vi "MainControl, FSM proto.vi"() -> ()   [LabVIEW 2020]
uses:
  State.ctl
panel:
  in  "Poll temps.":bool
  out "Repoll?":bool
  out "Current time":timestamp format="%<%X>T"
  out "Loop iteration":i32
  in  "Halt all":bool
  in  "Move dist.":dbl
  in  "Move up":bool
  in  "Move right":bool
  in  "Move left":bool
  in  "Move Down":bool
  in  "Home printer":bool
  in  "Stop print":bool
  out "STATE":T1
  in  "Start print":bool
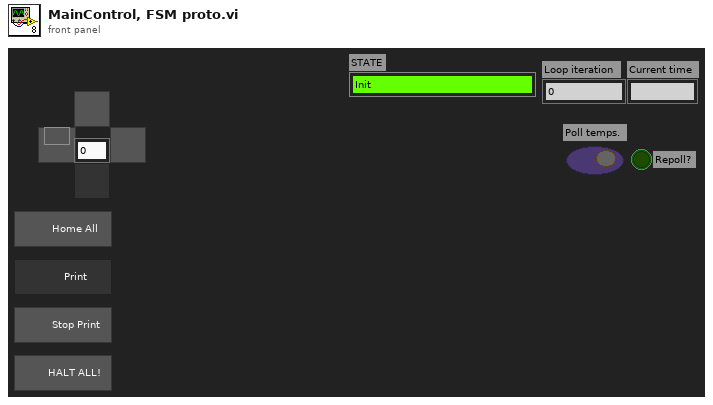
[diagram p1: front panel]
types:
  T1 = typedef "State.ctl" = enum16{"Init", "Idle", "Moving", "Printing - Container", "Printing - Curing", "Printing - Support Bath", "Printing - Biomaterial", "Stop print", "Halt all"}
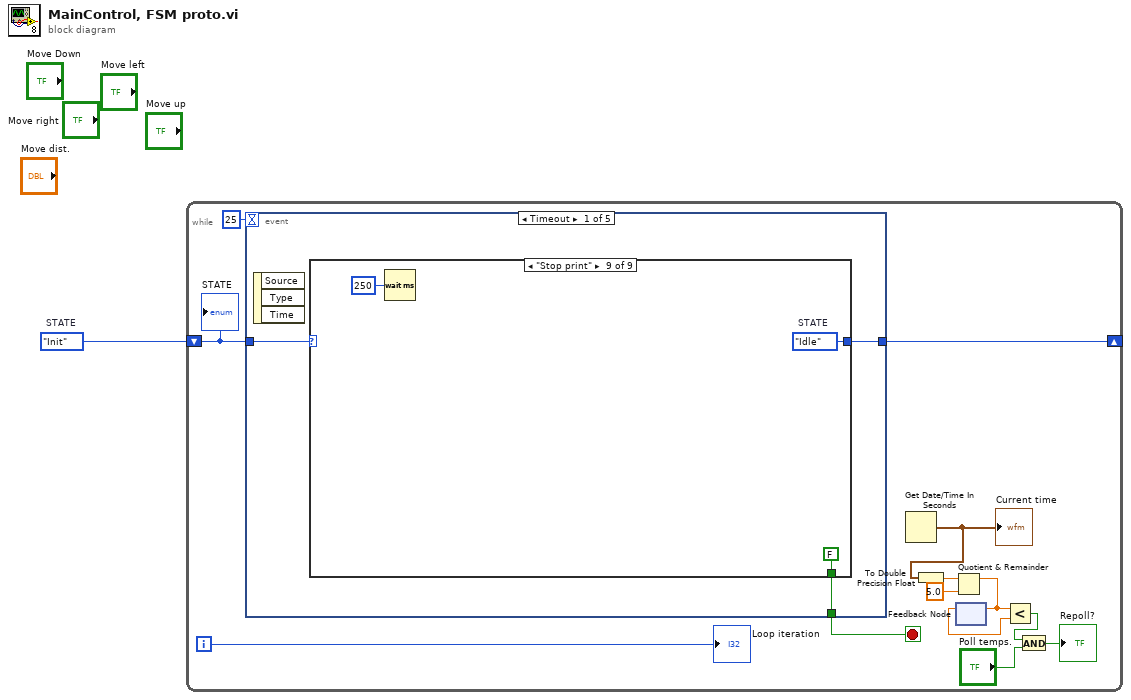
[diagram p0: block diagram]
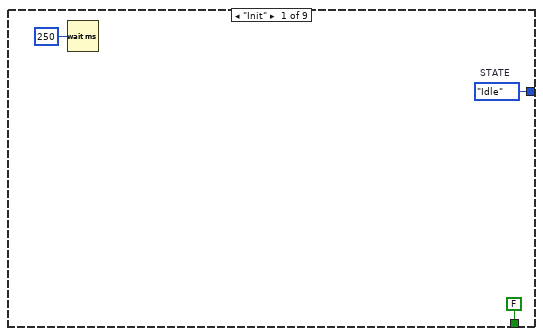
[diagram p2: hidden frame]
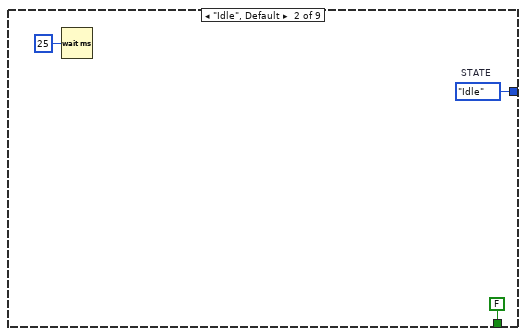
[diagram p3: hidden frame]
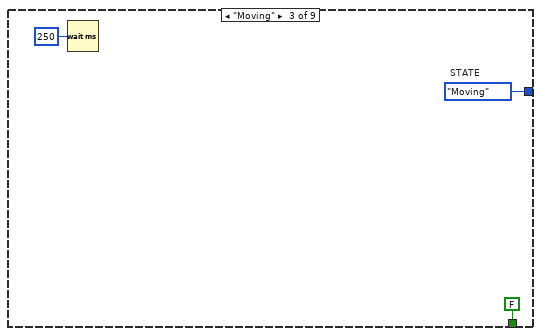
[diagram p4: hidden frame]
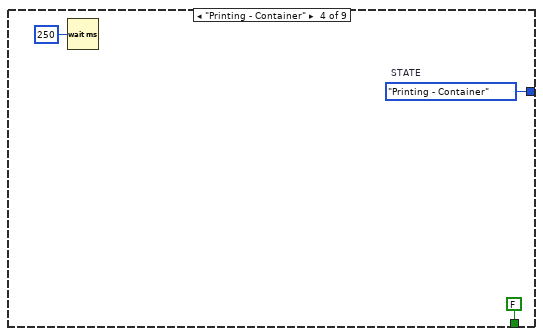
[diagram p5: hidden frame]
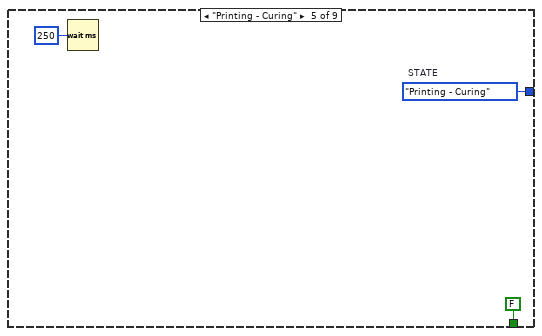
[diagram p6: hidden frame]
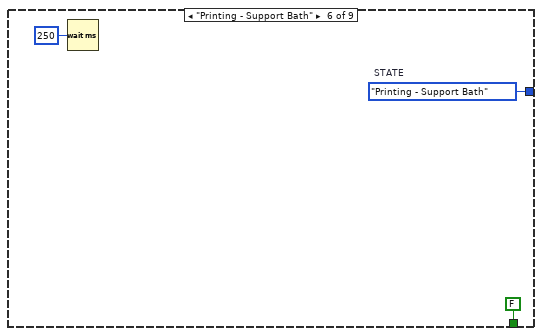
[diagram p7: hidden frame]
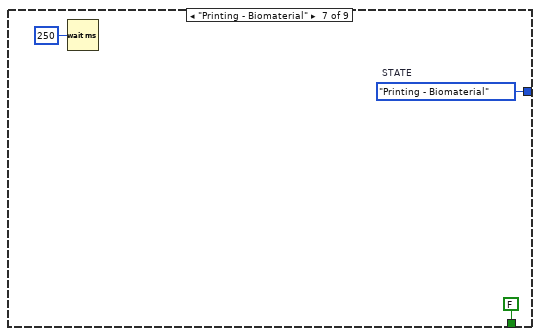
[diagram p8: hidden frame]
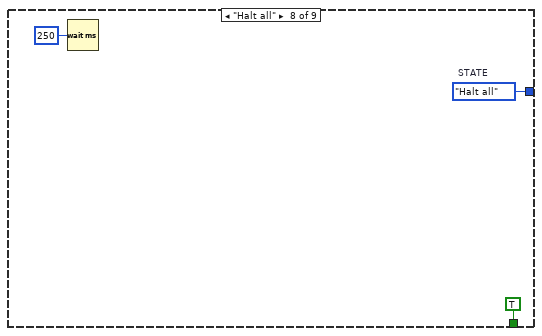
[diagram p9: hidden frame]
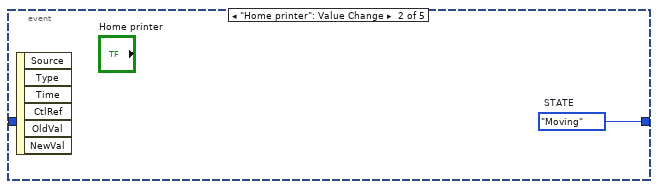
[diagram p10: hidden frame]
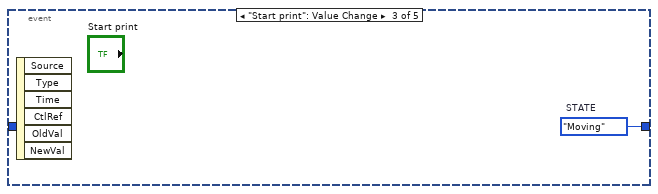
[diagram p11: hidden frame]
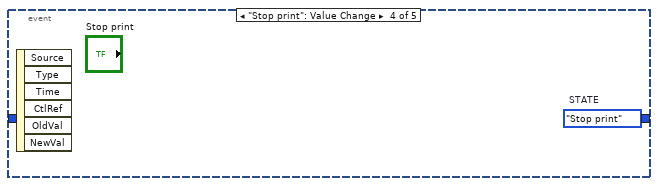
[diagram p12: hidden frame]
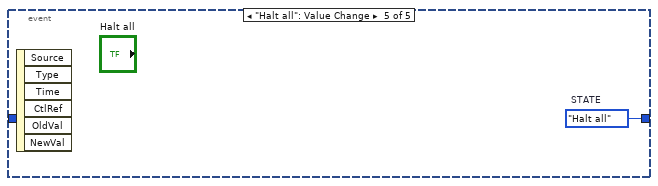
[diagram p13: hidden frame]
diagram:
  w1 = State."Init"  # STATE
  n1 = while {
    shift-right: [w12] -> _
    shift-left: w1 -> [w13]
    i -> [w10]
    stop <- w11 stop-if-true
    n2 = event shown="[0] Timeout" {
      selector: _ -> [_ _ _ _ _]
      dyn-events: _ -> [_ _ _ _ _]
      timeout: 25 -> [_ _ _ _ _]
      tunnel: w13 -> [w17 _ _ _ _]
      tunnel: [w16 w45 w46 w47 w48] -> w12
      tunnel: [w15 _ _ _ _] -> w11
      event Timeout {
        n3 = event-data() -> ()  [unwired: 1 in, 3 out]
        n4 = case shown="\"Stop print\"" w17 {
          tunnel: [w20 w23 w25 w29 w32 w35 w38 w41 w44] -> w16
          tunnel: [FALSE FALSE FALSE FALSE FALSE FALSE FALSE TRUE FALSE] -> w15
          frame "Init" {
            w20 = State."Idle"  # STATE
            n5 = Wait (ms)(milliseconds to wait=u32 250) -> ()  [unwired: 1 out]
          }
          frame "Idle", Default {
            w23 = State."Idle"  # STATE
            n6 = Wait (ms)(milliseconds to wait=u32 25) -> ()  [unwired: 1 out]
          }
          frame "Moving" {
            w25 = State."Moving"  # STATE
            n7 = Wait (ms)(milliseconds to wait=u32 250) -> ()  [unwired: 1 out]
          }
          frame "Printing - Container" {
            w29 = State."Printing - Container"  # STATE
            n8 = Wait (ms)(milliseconds to wait=u32 250) -> ()  [unwired: 1 out]
          }
          frame "Printing - Curing" {
            w32 = State."Printing - Curing"  # STATE
            n9 = Wait (ms)(milliseconds to wait=u32 250) -> ()  [unwired: 1 out]
          }
          frame "Printing - Support Bath" {
            w35 = State."Printing - Support Bath"  # STATE
            n10 = Wait (ms)(milliseconds to wait=u32 250) -> ()  [unwired: 1 out]
          }
          frame "Printing - Biomaterial" {
            w38 = State."Printing - Biomaterial"  # STATE
            n11 = Wait (ms)(milliseconds to wait=u32 250) -> ()  [unwired: 1 out]
          }
          frame "Halt all" {
            w41 = State."Halt all"  # STATE
            n12 = Wait (ms)(milliseconds to wait=u32 250) -> ()  [unwired: 1 out]
          }
          frame "Stop print" {
            w44 = State."Idle"  # STATE
            n13 = Wait (ms)(milliseconds to wait=u32 250) -> ()  [unwired: 1 out]
          }
        }
      }
      event "Home printer": Value Change {
        w45 = State."Moving"  # STATE
        n14 = event-data() -> ()  [unwired: 1 in, 6 out]
      }
      event "Start print": Value Change {
        w46 = State."Moving"  # STATE
        n15 = event-data() -> ()  [unwired: 1 in, 6 out]
      }
      event "Stop print": Value Change {
        w47 = State."Stop print"  # STATE
        n16 = event-data() -> ()  [unwired: 1 in, 6 out]
      }
      event "Halt all": Value Change {
        w48 = State."Halt all"  # STATE
        n17 = event-data() -> ()  [unwired: 1 in, 6 out]
      }
    }
    n18 = Get Date/Time In Seconds() -> (seconds since 1Jan1904=w7:timestamp)
    "Current time" <- w7
    n19 = To Double Precision Float(number=w7) -> (double precision float=w9:dbl)
    n20 = Quotient & Remainder(x=w9, y=5.0) -> (x-y*floor(x/y)=w5:dbl)  [unwired: 1 out]
    n21 = feedback #1() -> (w6:dbl)  [unwired: 1 in]
    n22 = feedback-in #1(w5) -> ()
    n23 = Less?(x=w5, y=w6) -> (x < y?=w4:bool)
    n24 = And(x=w4, y="Poll temps.") -> (x .and. y?=→"Repoll?":bool)
    "STATE" <- w13
    "Loop iteration" <- w10
  }
